vi "SPI_FPGA_Top_Level_Main_kyles.vi"(5 "FPGA IO":T1={"SCLK"="DIO18", "CS_1"="DIO16", "MOSI"="DIO26", "MISO"="DIO25"}) -> ()   [LabVIEW 2012]
uses:
  Controls/FPGA SPI_Cmd.ctl
  Controls/FPGA SPI_Arb Loop State.ctl
  <vilib>/rvi/eio/common/nirviEmuTemplateMethod_errors.vi
  <vilib>/rvi/Emulation/niFpgaSctlEmulationGetInTimedLoop.vi
  Code/FPGA SPI_Globals.vi
  <vilib>/rvi/Emulation/niFpgaSctlEmulationGlobalWrite.vi
  <vilib>/rvi/DataTransferAndStorage/Container/Common/niFpgaContainerGetUniqueNameForEmu.vi
  <vilib>/rvi/FIFO/Fifo_Resource/nirvififoEmulationSetSize.vi
  <vilib>/rvi/errors/niFpgaSetErrorForExecOnDevCompSimple.vi
  <vilib>/rvi/eio/common/nirviEmuReportErrorAndStop.vi
  <vilib>/rvi/Emulation/niFpgaSctlEmulationFifoFullMgr.vi
  <vilib>/rvi/Emulation/niFpgaSctlEmulationResourceMgr.vi
  <vilib>/eio/EIOMethodNode/EIOMethodNode.xnode
  <vilib>/eio/EIONode/EIONode.xnode
  <vilib>/rvi/DataTransferAndStorage/Container/XNode/niFpgaContainer.xnode
  <vilib>/rvi/FIFO/Fifo_Resource/nirvififoEmulationWrite.vi
  <vilib>/rvi/FIFO/Fifo_Resource/nirvififoEmulationRead.vi
panel:
  in  "SPI_Read?":bool
  out "Ready":bool
  in  "SPI_Clock Divider":u32=20
  in  "SPI_CS Active State":bool caption="SPI_CS\nActive State"
  in  "SPI_CPOL":bool
  in  "SPI_CPHA":bool
  in  "SPI_CS":u8=1 format="%08b"
  in  "SPI_Total Bits":u16=8
  in  "SPI_Total Bytes":u16=1
  in  "SPI_Start":bool
  in  "SPI_Cmd":T2=enum."Configure"
  in  "SPI_Ack Read":bool
  out "SPI_Read Data":u8
  out "SPI_Read Flag":bool
  in  "SPI_Write Flag":bool
  in  "SPI_Write Data":u8
  # "Control"
  # "SPI Configuration Parameters"
  # "Command Type"
  # "Host Data Transfer"
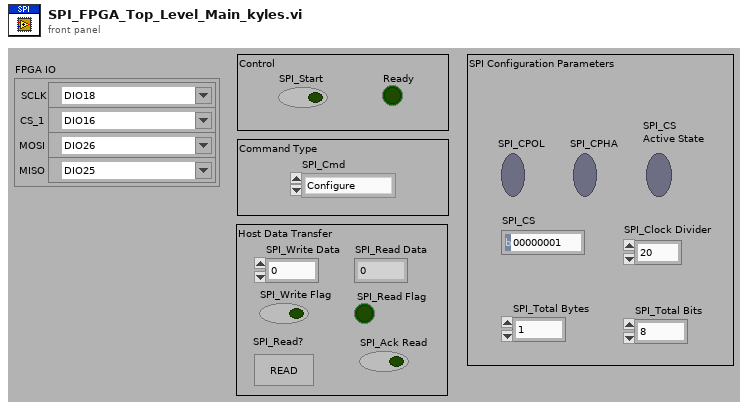
[diagram p1: front panel]
types:
  T1 = cluster{"SCLK":refnum<k21>, "CS_1":refnum<k21>, "MOSI":refnum<k21>, "MISO":refnum<k21>}
  T2 = typedef "FPGA SPI_Cmd.ctl" = enum8{"Idle", "Write/Read SPI", "Configure", "Restart"}
  T3 = enum16{"high", "wait", "low", "wait low", "high_2", "end"}
  T4 = typedef "FPGA SPI_Arb Loop State.ctl" = enum8{"Idle", "Init", "Write", "Start", "Read", "Wait Until Done"}
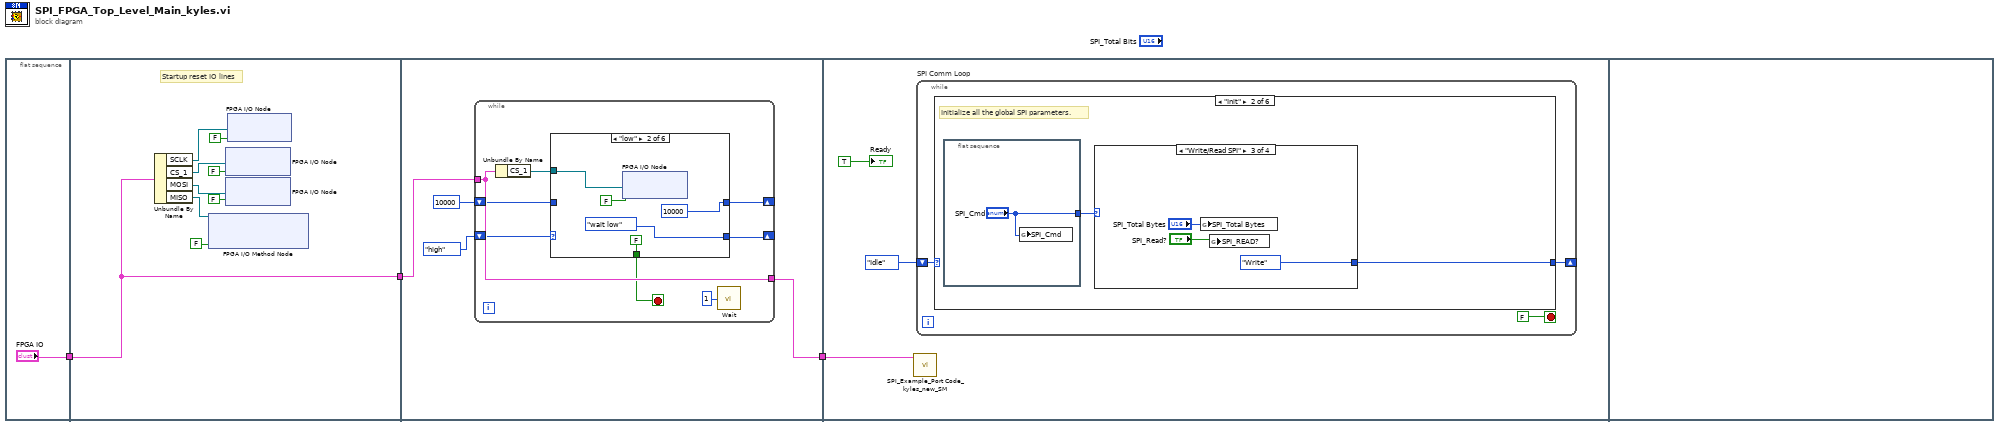
[diagram p0: block diagram]
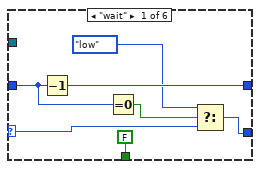
[diagram p2: hidden frame]
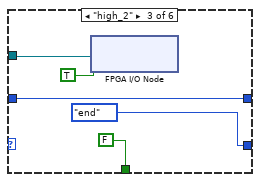
[diagram p3: hidden frame]
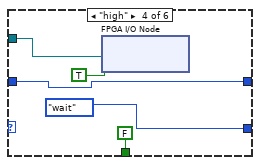
[diagram p4: hidden frame]
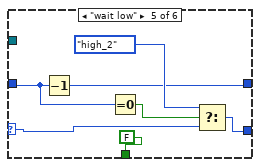
[diagram p5: hidden frame]
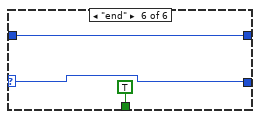
[diagram p6: hidden frame]
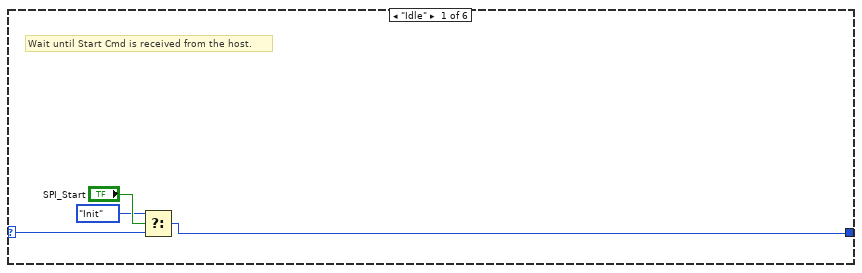
[diagram p7: hidden frame]
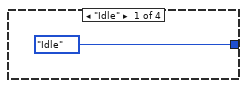
[diagram p8: hidden frame]
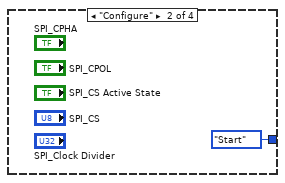
[diagram p9: hidden frame]
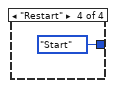
[diagram p10: hidden frame]
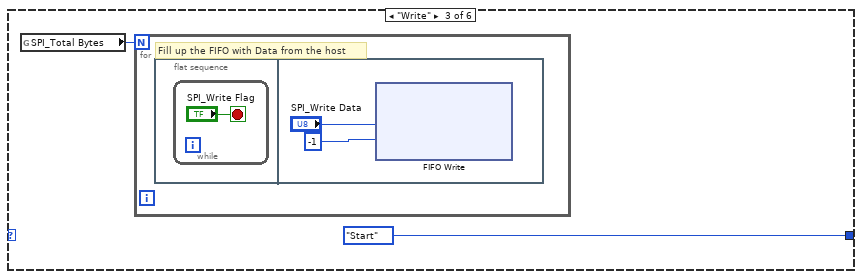
[diagram p11: hidden frame]
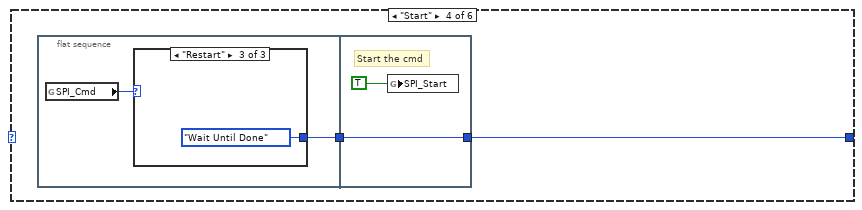
[diagram p12: hidden frame]
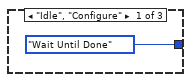
[diagram p13: hidden frame]
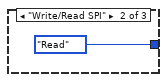
[diagram p14: hidden frame]
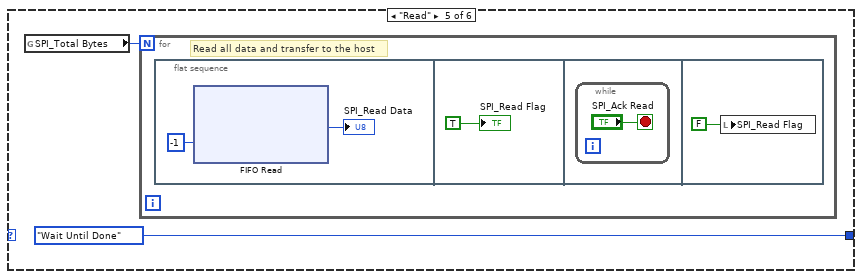
[diagram p15: hidden frame]
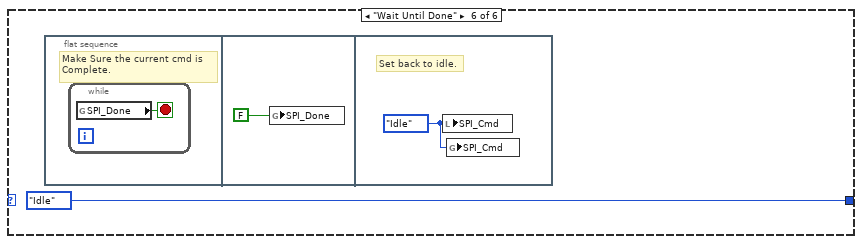
[diagram p16: hidden frame]
diagram:
  n1 = flat-sequence {
    tunnel: ["FPGA IO"] -> w3
    tunnel: w3 -> [w13]
    tunnel: [w13] -> w2
    tunnel: w2 -> [w17]
    tunnel: [w16] -> w1
    tunnel: w1 -> [w58]
    frame #0 {
    }
    frame #1 {
      # "Startup reset IO lines"
      n2 = Unbundle By Name(w13) -> ("SCLK"=w12:refnum<k21>, "CS_1"=w11:refnum<k21>, "MOSI"=w10:refnum<k21>, "MISO"=w5:refnum<k21>)
      n3 = xnode "FPGA I/O Method Node"("FPGA I/O In"=w5, "Enable"=FALSE) -> ()  [unwired: 1 out]
      n4 = xnode "FPGA I/O Node"("I/O Item"=FALSE, "FPGA I/O In"=w11) -> ()  [unwired: 1 out]
      n5 = xnode "FPGA I/O Node"("I/O Item"=FALSE, "FPGA I/O In"=w10) -> ()  [unwired: 1 out]
      n6 = xnode "FPGA I/O Node"("I/O Item"=FALSE, "FPGA I/O In"=w12) -> ()  [unwired: 1 out]
    }
    frame #2 {
      n7 = while {
        tunnel: w17 -> [w25]
        tunnel: [w25] -> w16
        shift-right: [w23] -> _
        shift-left: T3."high" -> [w22]
        shift-right: [w19] -> _
        shift-left: i16 10000 -> [w20]
        stop <- w21 stop-if-true
        n8 = Unbundle By Name(w25) -> ("CS_1"=w24:refnum<k21>)
        n9 = case shown="\"low\"" w22 {
          selector: w22 -> [w31 _ _ _ w50 w55]
          tunnel: w24 -> [_ w36 w39 w46 _ _]
          tunnel: [w30 T3."wait low" T3."end" T3."wait" w48 w55] -> w23
          tunnel: [FALSE FALSE FALSE FALSE FALSE TRUE] -> w21
          tunnel: w20 -> [w27 _ w41 w44 w51 w56]
          tunnel: [w29 i16 10000 w41 w44 w52 w56] -> w19
          frame "wait" {
            n10 = Decrement(x=w27) -> (x-1=w29:i16)
            n11 = Equal To 0?(x=w27) -> (x = 0?=w28:bool)
            n12 = Select(t=T3."low", s=w28, f=w31) -> (s? t:f=w30:T3)
          }
          frame "low" {
            n13 = xnode "FPGA I/O Node"("I/O Item"=FALSE, "FPGA I/O In"=w36) -> ()  [unwired: 1 out]
          }
          frame "high_2" {
            n14 = xnode "FPGA I/O Node"("I/O Item"=TRUE, "FPGA I/O In"=w39) -> ()  [unwired: 1 out]
          }
          frame "high" {
            n15 = xnode "FPGA I/O Node"("I/O Item"=TRUE, "FPGA I/O In"=w46) -> ()  [unwired: 1 out]
          }
          frame "wait low" {
            n16 = Decrement(x=w51) -> (x-1=w52:i16)
            n17 = Equal To 0?(x=w51) -> (x = 0?=w53:bool)
            n18 = Select(t=T3."high_2", s=w53, f=w50) -> (s? t:f=w48:T3)
          }
          frame "end" {
          }
        }
        n19 = call "Wait"("Count(Ticks)"=u8 1) -> ()  [unwired: 1 out]
      }
    }
    frame #3 {
      n20 = call "SPI_Example_Port Code_kyles_new_SM.vi"("FPGA IO"=w58) -> ()  [unwired: 11 in]
      n21 = while "SPI Comm Loop" {
        shift-right: [w62] -> _
        shift-left: FPGA_SPI_Arb_Loop_State."Idle" ("Action") -> [w61]
        stop <- FALSE stop-if-true
        n22 = case shown="\"Init\"" w61 {
          selector: w61 -> [w66 _ _ _ _ _]
          tunnel: [w64 w68 FPGA_SPI_Arb_Loop_State."Start" ("Action") w83 FPGA_SPI_Arb_Loop_State."Wait Until Done" ("Action") FPGA_SPI_Arb_Loop_State."Idle" ("Action")] -> w62
          frame "Idle" {
            # "Wait until Start Cmd is received from the host."
            n23 = Select(t=FPGA_SPI_Arb_Loop_State."Init" ("Action"), s="SPI_Start", f=w66) -> (s? t:f=w64:T4)
          }
          frame "Init" {
            # "Initialize all the global SPI parameters."
            n24 = flat-sequence {
              tunnel: ["SPI_Cmd"] -> w69
              frame #0 {
                n25 = global write "FPGA SPI_Globals.vi" "SPI_Cmd"("SPI_Cmd") -> ()
              }
            }
            n26 = case shown="\"Write/Read SPI\"" w69 {
              tunnel: [FPGA_SPI_Arb_Loop_State."Idle" ("Action") FPGA_SPI_Arb_Loop_State."Start" ("Action") FPGA_SPI_Arb_Loop_State."Write" ("Action") FPGA_SPI_Arb_Loop_State."Start" ("Action")] -> w68
              frame "Idle" {
              }
              frame "Configure" {
              }
              frame "Write/Read SPI" {
                n27 = global write "FPGA SPI_Globals.vi" "SPI_Total Bytes"("SPI_Total Bytes") -> ()
                n28 = global write "FPGA SPI_Globals.vi" "SPI_READ?"("SPI_Read?") -> ()
              }
              frame "Restart" {
              }
            }
          }
          frame "Write" {
            n29 = global read "FPGA SPI_Globals.vi" "SPI_Total Bytes"() -> (w78:u16)
            n30 = for {
              N: w78 -> [_]
              # "Fill up the FIFO with Data from the host"
              n31 = flat-sequence {
                frame #0 {
                  n32 = while {
                    stop <- "SPI_Write Flag" stop-if-true
                  }
                }
                frame #1 {
                  n33 = xnode ("FIFO Write")("Element"="SPI_Write Data", "Timeout"=-1) -> ()  [unwired: 1 in, 2 out]
                }
              }
            }
          }
          frame "Start" {
            n34 = flat-sequence {
              tunnel: [w84] -> w82
              tunnel: [w90] -> w83
              tunnel: w82 -> [w90]
              frame #0 {
                n35 = global read "FPGA SPI_Globals.vi" "SPI_Cmd"() -> (w85:T2)
                n36 = case shown="\"Restart\"" w85 {
                  tunnel: [FPGA_SPI_Arb_Loop_State."Wait Until Done" ("Action") FPGA_SPI_Arb_Loop_State."Read" ("Action") FPGA_SPI_Arb_Loop_State."Wait Until Done" ("Action")] -> w84
                  frame "Idle", "Configure" {
                  }
                  frame "Write/Read SPI" {
                  }
                  frame "Restart" {
                  }
                }
              }
              frame #1 {
                # "Start the cmd"
                n37 = global write "FPGA SPI_Globals.vi" "SPI_Start"(TRUE ("Write Flag")) -> ()
              }
            }
          }
          frame "Read" {
            n38 = global read "FPGA SPI_Globals.vi" "SPI_Total Bytes"() -> (w92:u16)
            n39 = for {
              N: w92 -> [_]
              # "Read all data and transfer to the host"
              n40 = flat-sequence {
                frame #0 {
                  n41 = xnode ("FIFO Read")("Timeout"=-1) -> ("Element"=→"SPI_Read Data":u8)  [unwired: 1 in, 2 out]
                }
                frame #1 {
                  "SPI_Read Flag" <- TRUE ("Read Flag")
                }
                frame #2 {
                  n42 = while {
                    stop <- "SPI_Ack Read" stop-if-true
                  }
                }
                frame #3 {
                  n43 = local write "SPI_Read Flag"(FALSE ("Read Flag")) -> ()
                }
              }
            }
          }
          frame "Wait Until Done" {
            n44 = flat-sequence {
              frame #0 {
                # "Make Sure the current cmd is\nComplete."
                n45 = while {
                  stop <- w99 stop-if-true
                  n46 = global read "FPGA SPI_Globals.vi" "SPI_Done"() -> (w99:bool)
                }
              }
              frame #1 {
                n47 = global write "FPGA SPI_Globals.vi" "SPI_Done"(FALSE ("Done")) -> ()
              }
              frame #2 {
                w101 = FPGA_SPI_Cmd."Idle" ("Type")
                # "Set back to idle."
                n48 = local write "SPI_Cmd"(w101) -> ()
                n49 = global write "FPGA SPI_Globals.vi" "SPI_Cmd"(w101) -> ()
              }
            }
          }
        }
      }
      "Ready" <- TRUE ("Ready")
    }
    frame #4 {
    }
  }
